vi "FTW-Endpoint-Multipart-Tell.vi"(0 "FTW Endpoint":refnum<class "FTW-Endpoint.lvclass">, 5 "Multipart Message":string[](array[string]), 7 "Timeout":i32 format="%dmsec", 11 "error in":errorcluster) -> (4 "FTW Endpoint out":refnum<class "FTW-Endpoint.lvclass">, 8 "Timed out?":bool, 15 "error out":errorcluster)   [LabVIEW 2012, in "FTW-Actor.lvlib" / "FTW-Endpoint.lvclass"]
uses:
  FTW-Endpoint.lvclass
  FTW-Endpoint.lvclass/FTW-Endpoint.ctl
panel:
  # "Inputs"
  # "Outputs"
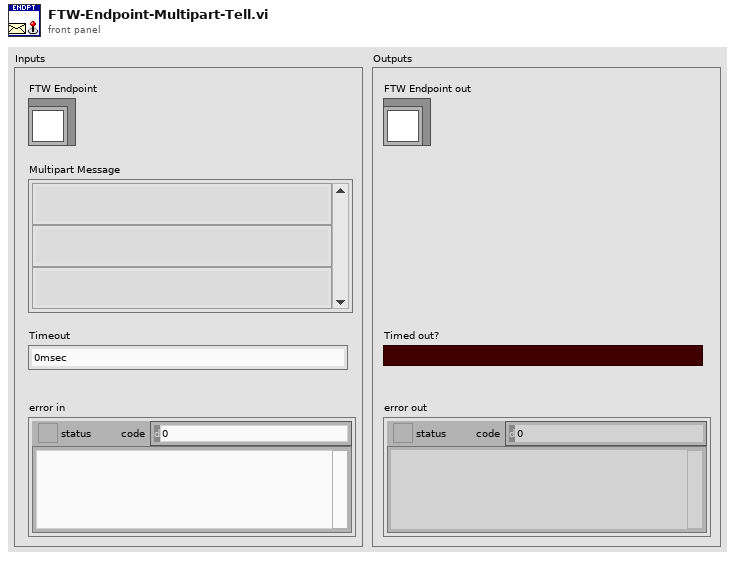
[diagram p1: front panel]
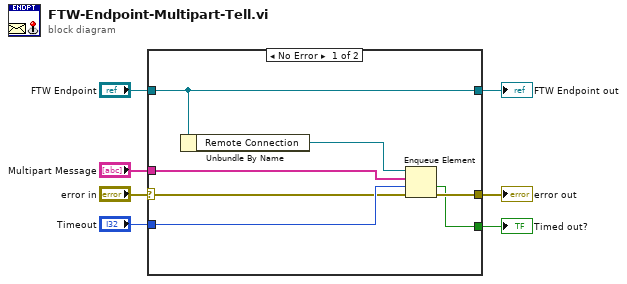
[diagram p0: block diagram]
diagram:
  n1 = case shown="No Error" "error in" {
    selector: "error in" -> [w8 w16]
    tunnel: [w14 w16] -> w7
    tunnel: [w10 w15] -> w5
    tunnel: "FTW Endpoint" -> [w10 w15]
    tunnel: "Multipart Message" -> [w11 _]
    tunnel: [w13 _] -> w2
    tunnel: "Timeout" -> [w12 _]
    frame No Error {
      n2 = Unbundle By Name(w10) -> ("Remote Connection"=w9:refnum<queue>)
      n3 = Enqueue Element(queue=w9, element=w11, timeout in ms (-1)=w12, error in (no error)=w8) -> (timed out?=w13:bool, error out=w14:errorcluster)  [unwired: 1 out]
    }
    frame Error {
    }
  }
  "error out" <- w7
  "FTW Endpoint out" <- w5
  "Timed out?" <- w2
